vi "niFPGA I32xI32 MAC+ MSB.vi"(5 "A":i32 format="%.0x", 7 "B":i32 format="%.0x", 9 "C":fxp<+/-,64,32> format="%.0x") -> (8 "A*B+C":i32=2838 format="%08x")   [LabVIEW 2017]
doc: "This utility VI implements a fractional 32 x 32 multiply and accumulate that returns a 32-bit result. It requires four 16 x 16 = 32 multipliers to compute the partial products, and adds in the accumulate value in parallel with the partial product adds to improve timing performance. \n\nThe output rounding mode is round to nearest (+Inf), and is achieved at no extra cost by incorporating the rounding bit into the accumulate add.\n\nThis VI does not handle overflow; it assumes the inputs are constrained to prevent overflow."
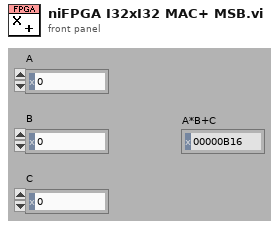
[diagram p1: front panel]
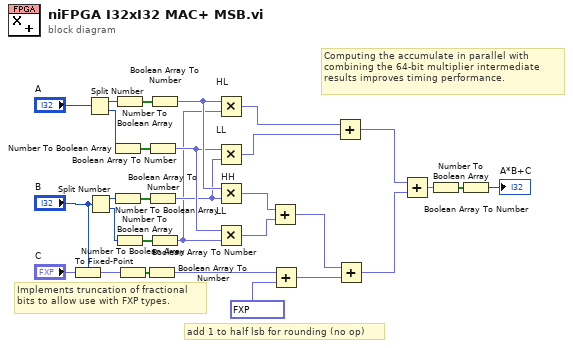
[diagram p0: block diagram]
diagram:
  # "add 1 to half lsb for rounding (no op)"
  # "Computing the accumulate in parallel with \ncombining the 64-bit multiplier intermediate \nresults improves timing performance."
  # "Implements truncation of fractional\nbits to allow use with FXP types."
  n1 = To Fixed-Point(fixed-point type="B", number="C") -> (fixed-point=w5:fxp<+/-,32,32>)
  n2 = Split Number(x="A") -> (hi(x)=w30:u16, lo(x)=w20:u16)
  n3 = Split Number(x="B") -> (hi(x)=w22:u16, lo(x)=w18:u16)
  n4 = Number To Boolean Array(number=w20) -> (Boolean array=w21:bool[])
  n5 = Number To Boolean Array(number=w22) -> (Boolean array=w23:bool[])
  n6 = Number To Boolean Array(number=w30) -> (Boolean array=w25:bool[])
  n7 = Number To Boolean Array(number=w18) -> (Boolean array=w19:bool[])
  n8 = Number To Boolean Array(number=w5) -> (Boolean array=w26:bool[])
  n9 = Boolean Array To Number(Boolean array=w26) -> (number=w15:fxp<+/-,32,0>)
  n10 = Boolean Array To Number(Boolean array=w21) -> (number=w12:fxp<+,16,-16>)
  n11 = Boolean Array To Number(Boolean array=w23) -> (number=w11:fxp<+/-,16,0>)
  n12 = Boolean Array To Number(Boolean array=w25) -> (number=w24:fxp<+/-,16,0>)
  n13 = Boolean Array To Number(Boolean array=w19) -> (number=w10:fxp<+,16,-16>)
  n14 = Multiply "HL"(x=w24, y=w10) -> (x*y=w16:fxp<+/-,32,-16>)
  n15 = Multiply "LL"(x=w12, y=w11) -> (x*y=w17:fxp<+/-,32,-16>)
  n16 = Multiply "HH"(x=w24, y=w11) -> (x*y=w28:fxp<+/-,32,0>)
  n17 = Multiply "LL"(x=w12, y=w10) -> (x*y=w27:fxp<+,32,-32>)
  n18 = Add(x=w28, y=w27) -> (x+y=w9:fxp<+/-,64,0>)
  n19 = Add(x=w15, y=fxp<+,1,-32> 1.1641532182693481e-10) -> (x+y=w13:fxp<+/-,33,0>)
  n20 = Add(x=w16, y=w17) -> (x+y=w8:fxp<+/-,33,-15>)
  n21 = Add(x=w9, y=w13) -> (x+y=w29:fxp<+/-,48,0>)
  n22 = Add(x=w8, y=w29) -> (x+y=w2:fxp<+/-,32,0>)
  n23 = Number To Boolean Array(number=w2) -> (Boolean array=w3:bool[])
  n24 = Boolean Array To Number(Boolean array=w3) -> (number=→"A*B+C":i32)
